vi "SwitchedDMM.vi"(4 "DMM ClassName":string="NI DMM4072.lvclass", 5 "Setting":T1={"Resolution (Digits)"=5.5, "Current Source (Amps)"=0.001, "Range"=2.0, "Measurement Type"=enum."DC Volts"} {"Resolution (Digits)" items=["3 1/2"=3.5, "4 1/2"=4.5, "5 1/2"=5.5, "6 1/2"=6.5, "7 1/2"=7.5]; "Current Source (Amps)" items=["1uA"=1e-06, "10uA"=1e-05, "100uA"=0.0001, "1mA"=0.001]}, 6 "DMM Ref":string="NI_DMM_4072", 7 "Connection(s)":string, 8 "error in":errorcluster, 9 "Switch Ref":string="NI_DMM_4072", 10 "Switch ClassName":string="NI DMM4072.lvclass", 11 "Base Path":path=path "C:/GitHub/OOP_OPC UA/Sequence/CodeModules/HAL/Concrete") -> (0 "error out":errorcluster={"status"=TRUE, "code"=-1073807346, "source"="VISA Open in APS-7000 Series.lvlib:Initialize.vi->Concrete.lvlib:APS7050.lvclass:Initialise.vi->Check objects.vi"}, 3 "Measurements":dbl)   [LabVIEW 2021]
uses:
  HAL/Harware Abstraction/Switch/Switch.lvclass
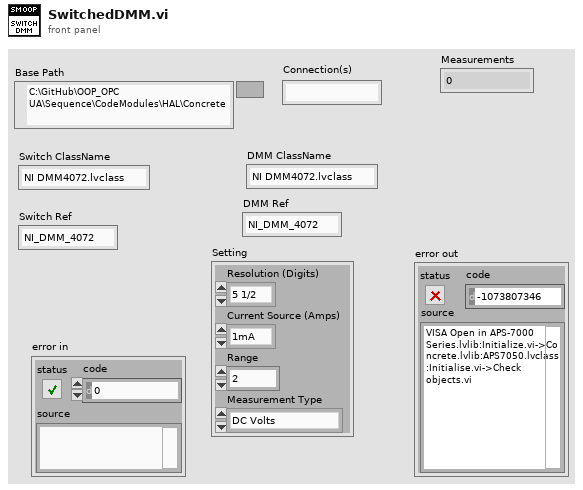
[diagram p1: front panel]
types:
  T1 = cluster{"Resolution (Digits)":dbl, "Current Source (Amps)":dbl, "Range":dbl, "Measurement Type":enum16{"DC Volts", "AC Volts", "DC Current", "AC Current", "2-wire Resistance", "4-wire Resistance", "Diode", "Frequency", "Period", "AC Volts DC Coupled", "Capacitance", "Inductance", "Temperature"}}
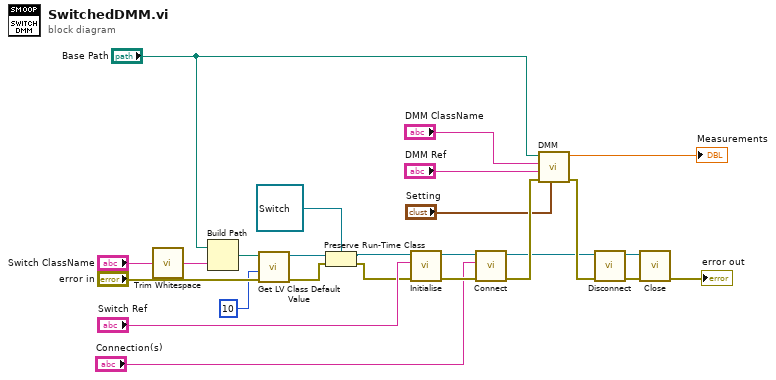
[diagram p0: block diagram]
diagram:
  n1 = call <vilib>:"Trim Whitespace.vi"("string"="Switch ClassName") -> ("trimmed string"=w23:string)  [unwired: 1 in]
  n2 = Build Path(base path="Base Path", name or relative path=w23) -> (appended path=w21:path)
  n3 = call <vilib>:"Get LV Class Default Value.vi"("error in (no error)"="error in", "options"=u32 10, "class path"=w21) -> ("error out"=w20:errorcluster, "object"=w24:refnum<class>)  [unwired: 7 in]
  n4 = Preserve Run-Time Class(object in=w24, error in=w20, 2:refnum<class "Switch.lvclass"> refnum ("HAL.lvlib:Switch.lvclass")) -> (object out=w18:refnum<class "Switch.lvclass">, error out=w17:errorcluster)
  n5 = call-dynamic "Initialise.vi"("error in (no error)"=w17, "Instrument Ref"="Switch Ref", "Instrument in"=w18) -> ("error out"=w14:errorcluster, "Instrument out"=w13:refnum<class "Switch.lvclass">)  [unwired: 7 in]
  n6 = call-dynamic "Connect.vi"("error in (no error)"=w14, "Channel(s)"="Connection(s)", "Switch in"=w13) -> ("error out"=w9:errorcluster, "Switch out"=w7:refnum<class "Switch.lvclass">)  [unwired: 7 in]
  n7 = call "DMM.vi"("Setting"="Setting", "error in"=w9, "DMM Ref"="DMM Ref", "DMM ClassName"="DMM ClassName", "Base Path"="Base Path") -> ("error out"=w8:errorcluster, "Measurements"=→"Measurements":dbl)  [unwired: 5 in]
  n8 = call-dynamic "Disconnect.vi"("error in (no error)"=w8, "Switch in"=w7) -> ("error out"=w12:errorcluster, "Switch out"=w11:refnum<class "Switch.lvclass">)  [unwired: 8 in]
  n9 = call-dynamic "Close.vi"("error in (no error)"=w12, "Instrument in"=w11) -> ("error out"=→"error out":errorcluster)  [unwired: 8 in, 1 out]
